vi "EdgeOff.vi"(11 "Current State":bool) -> (3 "Edge On Found":bool)   [LabVIEW 2020]
doc: "Edge On for general purpose\n\nInputs: Current state, Previous state\nFind a edge on.\nOutput: Edge on found (True) or not found (False)"
panel:
  out "Prior State":bool
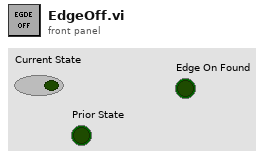
[diagram p1: front panel]
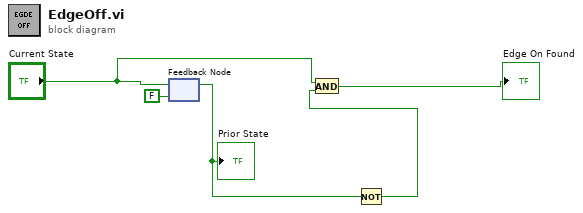
[diagram p0: block diagram]
diagram:
  n1 = feedback #1(FALSE ("Current State")) -> (w1:bool)
  "Prior State" <- w1
  n2 = feedback-in #1("Current State") -> ()
  n3 = Not(x=w1) -> (.not. x?=w3:bool)
  n4 = And(x="Current State", y=w3) -> (x .and. y?=→"Edge On Found":bool)
